vi "ReadRegisters.vi"(0 "Handle In":u64[](array[numeric]), 1 "error in (no error)":errorcluster, 5 "Device ID":u8=1, 7 "Read Start":u16=1, 9 "Read Amount":u16=16, 11 "Area":enum16{"Holding Registers", "Input Registers"}(ring)) -> (3 "error out":errorcluster, 4 "Handle Out":u64[](array[numeric]), 6 "Result":i32, 8 "RD Data":u16[](array[numeric]))   [LabVIEW 2020, in "SnapMB.lvlib"]
uses:
  SnapMB.lvlib
  windows/snapmb.dll
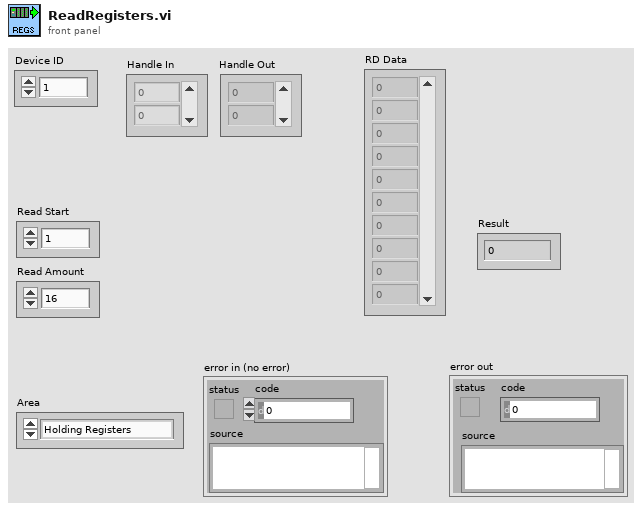
[diagram p1: front panel]
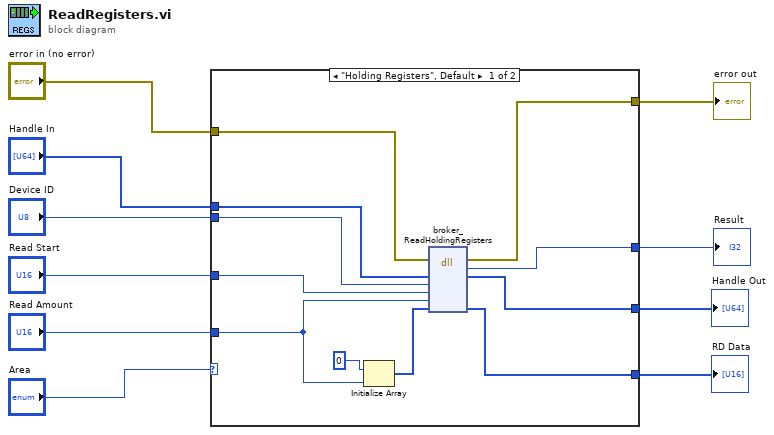
[diagram p0: block diagram]
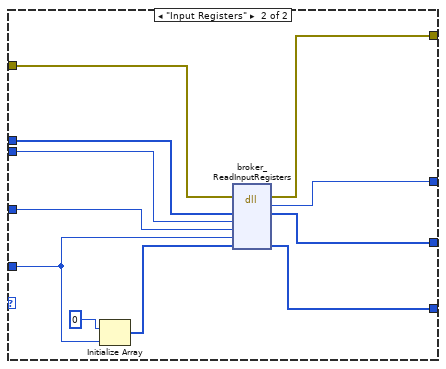
[diagram p2: hidden frame]
diagram:
  n1 = case shown="\"Holding Registers\", Default" "Area" {
    tunnel: "Handle In" -> [w16 w30]
    tunnel: "Device ID" -> [w17 w29]
    tunnel: "Read Start" -> [w18 w28]
    tunnel: "Read Amount" -> [w19 w26]
    tunnel: [w15 w24] -> w5
    tunnel: [w12 w23] -> w4
    tunnel: "error in (no error)" -> [w14 w32]
    tunnel: [w13 w31] -> w2
    tunnel: [w11 w22] -> w1
    frame "Holding Registers", Default {
      n2 = Initialize Array(u16 0 ("element"), w19) -> (w20:u16[])
      n3 = dll-call lib="D:/SnapMB/LabView/lib/windows/snapmb.dll" fn="broker_ReadHoldingRegisters"(error in=w14, "Handle"=w16, "DeviceID"=w17, "Start"=w18, "Amount"=w19, "pUsrData"=w20) -> (error out=w13:errorcluster, "Result"=w15:i32, "Handle"=w12:u64[], "pUsrData"=w11:u16[])  [unwired: 5 in, 1 out]
    }
    frame "Input Registers" {
      n4 = Initialize Array(u16 0 ("element"), w26) -> (w25:u16[])
      n5 = dll-call lib="D:/SnapMB/LabView/lib/windows/snapmb.dll" fn="broker_ReadInputRegisters"(error in=w32, "Handle"=w30, "DeviceID"=w29, "Start"=w28, "Amount"=w26, "pUsrData"=w25) -> (error out=w31:errorcluster, "Result"=w24:i32, "Handle"=w23:u64[], "pUsrData"=w22:u16[])  [unwired: 5 in, 1 out]
    }
  }
  "Result" <- w5
  "RD Data" <- w1
  "Handle Out" <- w4
  "error out" <- w2
